vi "图像属性.vi"() -> ()   [LabVIEW 2019]
uses:
  <vilib>/picture/cartesn2.llb/XY Plot Type.ctl
panel:
  in  "XY曲线修饰":T2(array[cluster])=[{"plot color"=16776960, "XY plot type"=enum."connected circles", "baseline"=0.0}, {"plot color"=65280, "XY plot type"=enum."connected circles", "baseline"=0.0}, {"plot color"=65535, "XY plot type"=enum."connected circles", "baseline"=0.0}, {"plot color"=16711680, "XY plot type"=enum."connected circles", "baseline"=0.0}]
  in  "尺寸（宽度、高度）":cluster{"width":i16, "height":i16}={"width"=900, "height"=700}
  in  "直角网格修饰":T3={"line color"=12369084, "text color"=16448250, "tick length(3)"=3, "crossing axes"=FALSE, "visible grid?"=TRUE}
  in  "直角坐标属性":T4={"x minimum"=0.0, "x maximum"=0.0, "x log?"=FALSE, "x precision"=2, "x format"=enum."Decimal", "y minimum"=0.0, "y maximum"=0.0, "y log?"=FALSE, "y precision"=1, "y format"=enum."Scientific"}
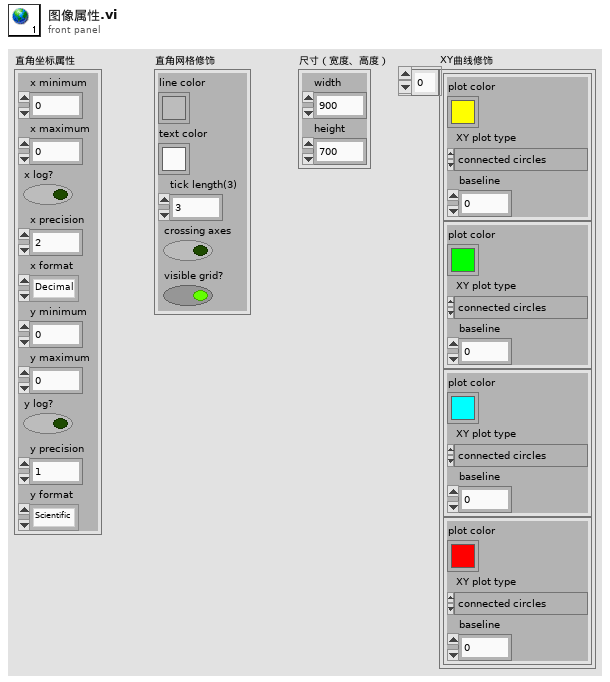
[diagram p1: front panel]
types:
  T1 = typedef "XY Plot Type.ctl" = enum16{"points", "squares", "circles", "connected points", "connected squares", "connected circles", "comb plot", "sized scatter plot", "sized-colored scatter plot", "min-max lines"}
  T2 = cluster{"plot color":u32, "XY plot type":T1, "baseline":dbl}[]
  T3 = cluster{"line color":u32, "text color":u32, "tick length(3)":i16, "crossing axes":bool, "visible grid?":bool}
  T4 = cluster{"x minimum":dbl, "x maximum":dbl, "x log?":bool, "x precision":u8, "x format":enum8{"Decimal", "Scientific", "Engineering", "Binary", "Octal", "Hex"}, "y minimum":dbl, "y maximum":dbl, "y log?":bool, "y precision":u8, "y format":enum8{"Decimal", "Scientific", "Engineering", "Binary", "Octal", "Hex"}}
diagram:
